vi "Fetch U8 data.vi"(4 "error in (no error)":errorcluster, 7 "Statement Refnum":T1) -> (0 "error out":errorcluster, 2 "Data":u8, 3 "Statement Refnum":T1)   [LabVIEW 2011]
doc: "Lit la donnée de type entier (I16)"
uses:
  SQL Controls/Statement Refnum.ctl
  Odbc32.dll
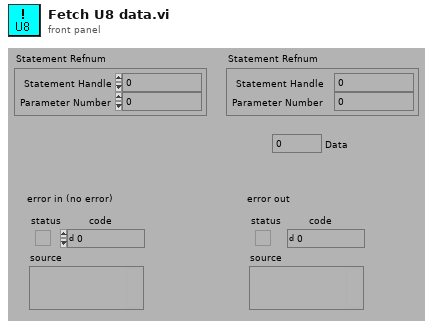
[diagram p1: front panel]
types:
  T1 = typedef "Statement Refnum.ctl" = cluster{"Statement Handle":i32, "Parameter Number":u16}
  T2 = enum16{"NOPE", "SQL_HANDLE_ENV", "SQL_HANDLE_DBC", "SQL_HANDLE_STMT", "SQL_HANDLE_DESC"}
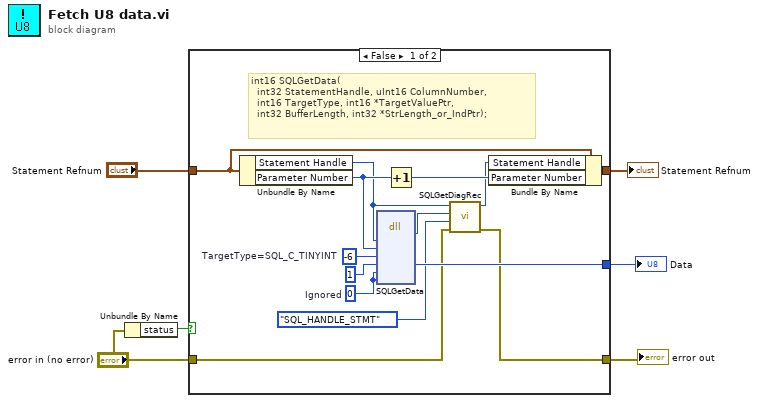
[diagram p0: block diagram]
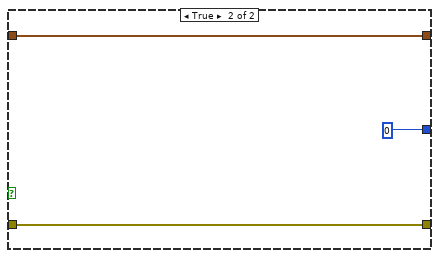
[diagram p2: hidden frame]
diagram:
  n1 = Unbundle By Name("error in (no error)") -> ("status"=w1:bool)
  n2 = case shown="False" w1 {
    tunnel: [w20 u8 0] -> w6
    tunnel: "Statement Refnum" -> [w19 w22]
    tunnel: [w18 w22] -> w4
    tunnel: [w11 w23] -> w3
    tunnel: "error in (no error)" -> [w10 w23]
    frame False {
      w15 = i16 -6  # TargetType=SQL_C_TINYINT
      w8 = 0  # Ignored
      # "int16 SQLGetData(\n  int32 StatementHandle, uInt16 ColumnNumber, \n  int16 TargetType, int16 *TargetValuePtr,\n  int32 BufferLength, int32 *StrLength_or_IndPtr);"
      n3 = Unbundle By Name(w19) -> ("Statement Handle"=w13:i32, "Parameter Number"=w17:u16)
      n4 = dll-call lib="Odbc32.dll" fn="SQLGetData"("StatementHandle"=w13, "ColumnNumber"=w17, "TargetType"=w15, "TargetValuePtr"=u8 1, "BufferLength"=w8, "StrLength_or_IndPtr"=w8) -> (w14:i16, "TargetValuePtr"=w20:u8)  [unwired: 7 in, 3 out]
      n5 = Increment(x=w17) -> (x+1=w16:u16)
      n6 = call "SQLGetDiagRec.vi"("error in (no error)"=w10, "HandleType"=T2."SQL_HANDLE_STMT", "Status (SQL_SUCCESS=0)"=w14, "Input Handle"=w13) -> ("error out"=w11:errorcluster, "Output Handle"=w12:i32)  [unwired: 2 out]
      n7 = Bundle By Name(cluster=w19, "Statement Handle"=w12, "Parameter Number"=w16) -> (w18:T1)
    }
    frame True {
    }
  }
  "Statement Refnum" <- w4
  "Data" <- w6
  "error out" <- w3
